vi "Color Matching.vi"() -> ()   [LabVIEW 2014]
doc: "This example shows how to use IMAQ ColorMatch to check LEDs on the front panel of an instrument. This example compares the color inside each region of interest (ROI) that surrounds an LED to the color spectrum of the expected color. The VI uses another example to learn the color spectrums."
uses:
  <vilib>/vision/NI_Vision_Development_Module.lvlib
panel:
  in  "Stop":bool
  out "Expected Pattern":T1
  out "Pass/Fail":T2
  in  "Orange Color Array":u32[][](array[colorbox])=[[14251822, 15569449, 16163116, 16492861, 15505723, 14721096, 14458954, 14263380, 14134114, 13741935, 13546876, 13746316, 14207641, 14539441, 13355173], [16488515, 16227377, 16163374, 16625472, 15902529, 15972181, 15775833, 15514209, 15253100, 14663027, 14401406, 14600845, 15259037, 15854523, 14078888], [16357434, 16293942, 15900982, 15574075, 15575618, 14328890, 14394944, 14527565, 14463835, 14201958, 14006129, 14336385, 14863504, 13813911, 14077859], [15634981, 16361273, 15903040, 14523444, 14525240, 14658112, 14527557, 14659921, 14858593, 14793838, 14597496, 14861446, 15322258, 14536867, 15393208], [15637012, 16494389, 16365383, 15315266, 15317058, 15118924, 14790476, 14659668, 14660961, 14661741, 14530424, 14596993, 14794891, 13681048, 14668464], [16756504, 15903782, 15051057, 14593334, 14529588, 14922316, 14527819, 14264912, 14462814, 14464110, 14530425, 14662277, 14925709, 14996142, 14010023], [16163605, 15442980, 14393902, 14529592, 14334002, 14265926, 14003015, 13871694, 14069083, 14135143, 14267253, 14728070, 15319954, 14534051, 14272166], [16163860, 15377187, 14130730, 14002480, 13412901, 14331972, 14069060, 14003533, 14135128, 14069861, 14201457, 14530943, 14991755, 14007703, 14338212], [16032531, 15706152, 14787891, 14462263, 13872171, 14463809, 14331972, 14201164, 14398553, 14267491, 14070892, 14399865, 14729349, 14600604, 15127724], [16032532, 15969326, 15313724, 15184961, 14528820, 14529087, 14397761, 14332746, 14399321, 14399588, 14202989, 14335353, 14664578, 14929567, 15062184], [16032795, 15968560, 15246650, 14986301, 14264621, 14265918, 14134593, 14135371, 14333274, 14268774, 14203506, 14401661, 14730889, 14469016, 14272668], [15834913, 15770930, 15114553, 14919995, 14263595, 14264898, 14002756, 14003534, 14136157, 14137196, 14138489, 14402439, 14797714, 14864293, 14799531], [15768871, 16033338, 15508544, 15576898, 14986802, 14659151, 14396496, 14331994, 14399080, 14400119, 14466949, 14665876, 15192480, 15456182, 15654335], [15965997, 16296256, 15705923, 15708484, 15183668, 15251037, 14988383, 14792295, 14793588, 14663554, 14730640, 15126176, 15587501, 14600620, 15061947], [14516283, 15768133, 16493647, 16561234, 16167503, 14856808, 14922862, 15056509, 15189902, 14928280, 14272669, 14142373, 14274989, 12501671, 11580573]]
  in  "Red Color Array":u32[][](array[colorbox])=[[12910680, 13959787, 15404161, 16651920, 16717199, 16650119, 16385925, 15992448, 16061061, 16329616, 16269977, 15948193, 16415413, 16750539, 15770563], [14225000, 15076985, 16061062, 16651407, 16716171, 16386947, 16453001, 16059268, 15996549, 16132749, 15678608, 15158677, 15296673, 15958452, 16032967], [15406707, 16127876, 16388746, 16453515, 16322183, 16059009, 16718994, 16588176, 16721812, 16726941, 16665503, 16079777, 16019626, 16417974, 15703489], [16128123, 16718219, 16585614, 16454287, 16323982, 16258957, 15932815, 15999119, 16329877, 16727453, 16403871, 15883168, 15690661, 15890860, 15505083], [16718470, 16718994, 16718232, 16653466, 16590240, 16592035, 16728495, 16729007, 16731058, 16734389, 16737205, 16739507, 16545972, 16417207, 15437750], [16652939, 16718746, 16719009, 16524711, 16396974, 16333232, 15942063, 16073902, 16403119, 16667569, 16670643, 16477107, 16151989, 15891638, 15173295], [16389775, 16653214, 16720811, 16593334, 16268989, 15811516, 16077760, 16274880, 16669121, 16736448, 16739780, 16743625, 16746443, 16747978, 15238577], [16390806, 16720551, 16723897, 16728519, 16600524, 16011465, 16342989, 16539851, 16539590, 16540354, 16607938, 16676804, 16417222, 16221381, 15961786], [16191618, 16654236, 16726711, 16730560, 16601794, 16735945, 16735693, 16736204, 16736711, 16475331, 16215231, 16086977, 16221381, 16354761, 16361936], [16717714, 16720294, 16726206, 16466885, 16075203, 16535750, 16538054, 16669636, 16670659, 16541376, 16346815, 16415682, 16484294, 16617674, 14913207], [16322191, 16719017, 16726216, 16730835, 16733142, 16735451, 16406977, 16538562, 16670913, 16606398, 16345786, 16217274, 16219323, 16155580, 15371705], [16586125, 16719781, 16725181, 16466117, 16401862, 16732365, 16669891, 16736196, 16737473, 16739009, 16740541, 16611260, 16482235, 16483516, 15371191], [16456322, 16721051, 16724654, 16333234, 16268722, 16730300, 15550127, 15813553, 16143025, 16276404, 16213170, 16084659, 16086964, 16022965, 15240119], [15799920, 16654988, 16724644, 16660395, 16726955, 16729779, 16732863, 16734146, 16735682, 16737473, 16739775, 16676542, 16482238, 16352959, 15505344], [15209577, 15997828, 16591004, 16395169, 16066202, 16656797, 16006064, 16072622, 16074415, 15879853, 15488939, 15229611, 15035821, 14972079, 14981823]]
  in  "Green Color Array":u32[][](array[colorbox])=[[5534475, 8890654, 10009630, 10535962, 10536465, 9812224, 9218821, 9415686, 9612811, 9809426, 9809179, 9873705, 9873205, 10069565, 10265687], [8562206, 10076183, 10405390, 9878533, 9351424, 9219584, 9482498, 9942279, 10337037, 10665238, 10664737, 10532138, 10136626, 10004021, 10200145], [9879321, 10209026, 10668801, 10338305, 9745152, 10337289, 9877506, 10403080, 10929426, 11257626, 11388710, 11321907, 10794807, 10399030, 10266189], [10340626, 9814272, 10471168, 10337792, 9744896, 10731021, 10469389, 11061012, 11455770, 11783971, 12046642, 12243009, 11847495, 11320134, 10792533], [10538258, 9616640, 10207232, 10008320, 9546496, 10467073, 10666519, 11257886, 11586851, 11783467, 12243516, 12703055, 12439383, 11845973, 10792282], [9880075, 9747712, 10469640, 10731275, 10796038, 11650829, 10797602, 11455018, 11717936, 11849012, 12374855, 12965979, 12636261, 11911519, 11120996], [10274581, 10470418, 10731796, 10533646, 10466819, 11124482, 11192111, 11849271, 12178236, 12309059, 12769108, 13360233, 12964975, 12174186, 12173688], [10733841, 10338567, 10074633, 10073101, 10007049, 10336267, 10336804, 11060273, 11783743, 12046665, 12243796, 12309086, 12111204, 11716195, 11583857], [10010883, 9812480, 9810944, 9678594, 10073095, 11059216, 11454766, 11717683, 11980859, 12112194, 12440656, 12703327, 12571238, 12242022, 12306810], [10274308, 10602240, 10732549, 10205443, 10269954, 10993163, 11257890, 11455015, 11652397, 11783478, 12046149, 12308819, 12110939, 11584344, 12306810], [10537738, 10799872, 10798592, 10599938, 10532864, 10730243, 11521052, 11981349, 12507442, 12704318, 12835403, 12900696, 12637024, 12176223, 11779955], [10405653, 9747712, 9614336, 10336256, 10730243, 10992388, 10008064, 10599948, 11126041, 11125540, 11124785, 11255873, 11320910, 11254868, 11714166], [10076451, 10207497, 10272000, 10664963, 10663682, 10531584, 10928653, 11257365, 11322909, 11125029, 11190068, 11649867, 12043869, 12175206, 11450230], [8693794, 10733341, 11587354, 11256336, 10465793, 10399488, 10204931, 10204679, 10072590, 10137883, 10597680, 10991686, 10925139, 10529878, 9476189], [6324746, 9614357, 11389212, 10795533, 10399748, 11385616, 9809152, 9743105, 9808651, 10334240, 11123004, 11253838, 10331982, 9147461, 7172414]]
  in  "Black Color Array":u32[][](array[colorbox])=[[66055, 66055, 66055, 66055, 66055, 66055, 66055, 66055, 66055, 66055, 66055, 66055, 66055, 66055, 66054], [65803, 65803, 65803, 65803, 65803, 65803, 66055, 66055, 66055, 66055, 66055, 66055, 66055, 66055, 66054], [65803, 65803, 65803, 65803, 65803, 65803, 66055, 66055, 66055, 66055, 66055, 66055, 66055, 66055, 66054], [65803, 65803, 65803, 65803, 65803, 65803, 66055, 66055, 66055, 66055, 66055, 66055, 66055, 66055, 66054], [65801, 65801, 65801, 65801, 65801, 65801, 66055, 66055, 66055, 66055, 66055, 66055, 66055, 66055, 66054], [65801, 65801, 65801, 65801, 65801, 65801, 66055, 66055, 66055, 66055, 66055, 66055, 66055, 66055, 66054], [65803, 65803, 65803, 65803, 65803, 65803, 66055, 66055, 66055, 66055, 66055, 66055, 66055, 66055, 66054], [65803, 65803, 65803, 65803, 65803, 65803, 66055, 66055, 66055, 66055, 66055, 66055, 66055, 66055, 66054], [65803, 65803, 65803, 65803, 65803, 65803, 66055, 66055, 66055, 66055, 66055, 66055, 66055, 66055, 66054], [66055, 66055, 66055, 66055, 66055, 66055, 66306, 66306, 66306, 66306, 66306, 66306, 66306, 66306, 66306], [66055, 66055, 66055, 66055, 66055, 66055, 66306, 66306, 66306, 66306, 66306, 66306, 66306, 66306, 66306], [65801, 65801, 65801, 65801, 65801, 65801, 66306, 66306, 66306, 66306, 66306, 66306, 66306, 66306, 66306], [131594, 131594, 131594, 131594, 131594, 131594, 66052, 66052, 66052, 66052, 66052, 66052, 66052, 66052, 66306], [131596, 131596, 131596, 131596, 131596, 131596, 66052, 66052, 66052, 66052, 66052, 66052, 66052, 66052, 66306], [197389, 197389, 197389, 197389, 197389, 197389, 66054, 66054, 66054, 66054, 66054, 66054, 66054, 66054, 66306]]
  out "Color Image":T3(plugin-control)
  out "Orange Color Spectrum":dbl[][](graph)
  out "Red Color Spectrum":dbl[][](graph)
  in  "Delay (s.)":dbl(slide)=0.9859154929577465 scale=0.0..3.0
  out "Black Color Spectrum":dbl[][](graph)
  out "Global Status":bool=TRUE
  out "Green Color Spectrum":dbl[][](graph)
  # "Overview: Demonstrates how to use the IMAQ Color Learn function to create a color spectrum array which is used by the IMAQ ColorMatch function to verify the LED has the expected color.\nRequirements: Vision Development Software.\nInstructions:  Run the VI."
  # "Faults"
  # "Inhibits"
  # "Limits"
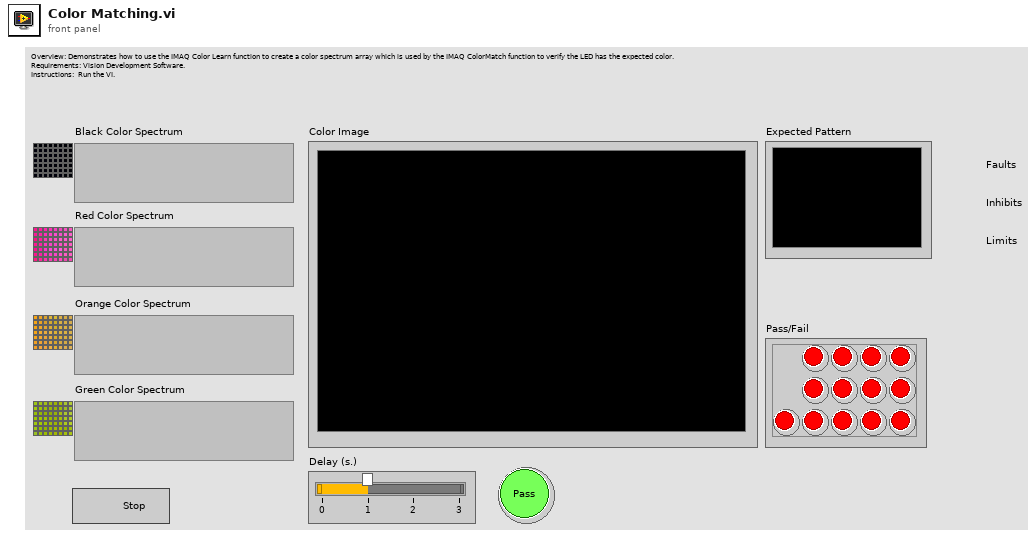
[diagram p1: front panel]
types:
  T1 = cluster{"on/off":i32, "Fault 1":i32, "Fault 2":i32, "Fault 3":i32, "Fault 4":i32, "Inhibit 1":i32, "Inhibit 2":i32, "Inhibit 3":i32, "Inhibit 4":i32, "Limit 1":i32, "Limit 2":i32, "Limit 3":i32, "Limit 4":i32}
  T2 = cluster{"Fault 2":bool, "Fault 1":bool, "Fault 3":bool, "Fault 4":bool, "Fault 5":bool, "Fault 6":bool, "Fault 7":bool, "Fault 8":bool, "Fault 9":bool, "Fault 10":bool, "Fault 11":bool, "Fault 12":bool, "Fault 13":bool}
  T3 = typedef "IMAQ Image.ctl" = refnum<image>
  T4 = cluster{"Global Rectangle":i32[], "Contours":cluster{"ID":enum32{"External", "Internal"}, "Type":u32, "Coordinates":i32[]}[]}[]
  T5 = cluster{"on/off":i32, "Fault 1":i32, "Fault 2":i32, "Fault 3":i32, "Fault 4":i32, "Inhibit 1":i32, "Inhibit 2":i32, "Inhibit 3":i32, "Inhibit 4":i32, "Limit 1":i32, "Limit 2":i32, "Limit 3":i32, "Limit 4":i32}[]
  T6 = typedef "Image Type" = u32
  T7 = cluster{"Desired Font (Application)":enum16{"User-specified Font", "Application Font", "System Font", "Dialog Font"}, "[User-specified Font]":cluster{"Font Name":string, "Size":i16, "Strikeout?":bool, "Italic?":bool, "Underline?":bool, "Outline?":bool, "Shadow?":bool, "Bold?":bool, "Rotation Angle":dbl}, "Horizontal Alignment":i16, "Vertical Alignment":i16}
  T8 = cluster{"Global Rectangle[0]":i32, "Global Rectangle[1]":i32}
  T9 = cluster{"[0]":bool, "[1]":bool, "[2]":bool, "[3]":bool, "[4]":bool, "[5]":bool, "[6]":bool, "[7]":bool, "[8]":bool, "[9]":bool, "[10]":bool, "[11]":bool, "[12]":bool}
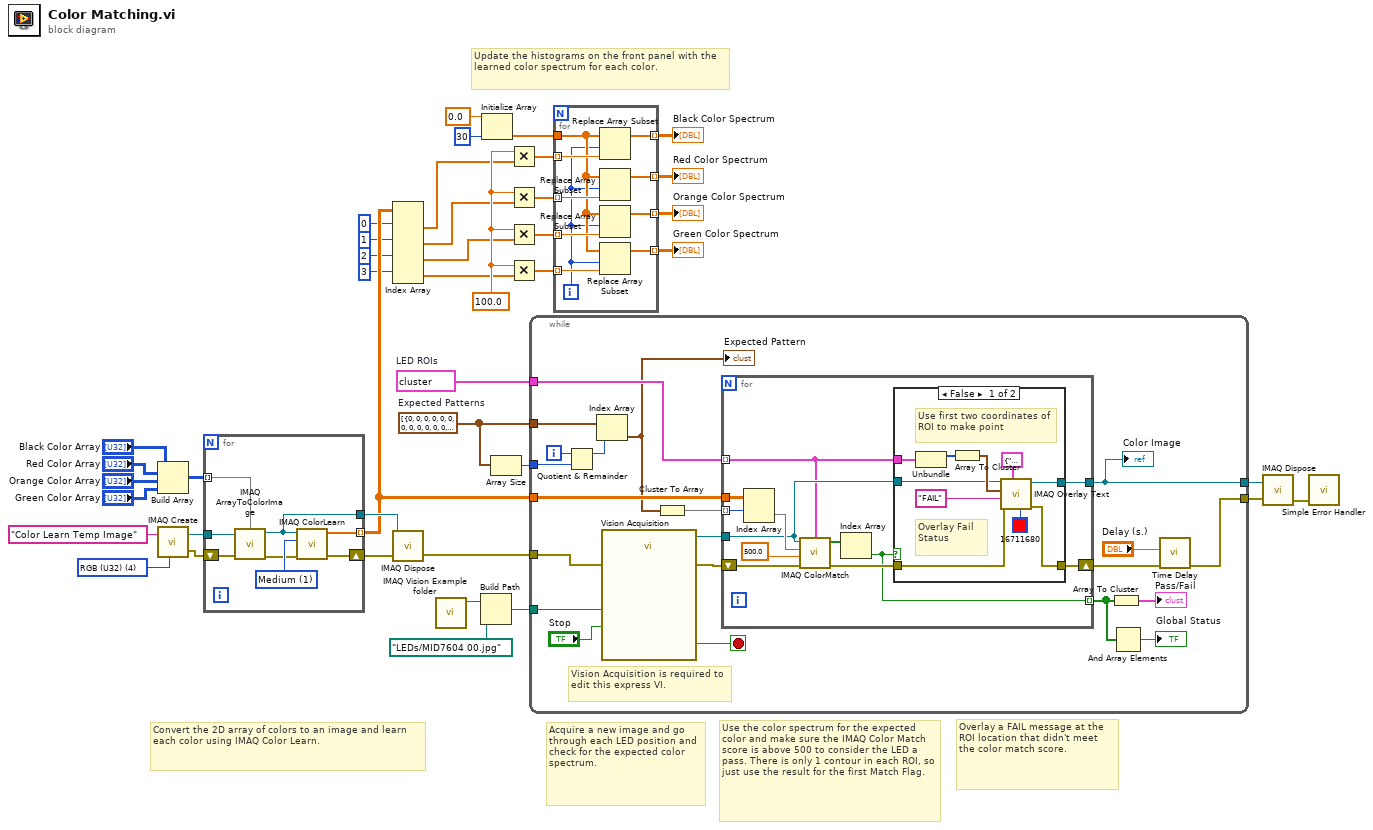
[diagram p0: block diagram]
diagram:
  w12 = T4 [{"Global Rectangle"=[32, 224, 53, 245], "Contours"=[{"ID"=enum."External", "Type"=3, "Coordinates"=[32, 224, 53, 245]}]}, {"Global Rectangle"=[86, 154, 98, 166], "Contours"=[{"ID"=enum."External", "Type"=3, "Coordinates"=[86, 154, 98, 166]}]}, {"Global Rectangle"=[136, 153, 149, 167], "Contours"=[{"ID"=enum."External", "Type"=3, "Coordinates"=[136, 153, 149, 167]}]}, {"Global Rectangle"=[188, 152, 200, 167], "Contours"=[{"ID"=enum."External", "Type"=3, "Coordinates"=[188, 152, 200, 167]}]}, {"Global Rectangle"=[236, 152, 250, 168], "Contours"=[{"ID"=enum."External", "Type"=3, "Coordinates"=[236, 152, 250, 168]}]}, {"Global Rectangle"=[87, 194, 99, 207], "Contours"=[{"ID"=enum."External", "Type"=3, "Coordinates"=[87, 194, 99, 207]}]}, {"Global Rectangle"=[136, 193, 149, 208], "Contours"=[{"ID"=enum."External", "Type"=3, "Coordinates"=[136, 193, 149, 208]}]}, {"Global Rectangle"=[189, 193, 201, 207], "Contours"=[{"ID"=enum."External", "Type"=3, "Coordinates"=[189, 193, 201, 207]}]}, {"Global Rectangle"=[236, 194, 250, 208], "Contours"=[{"ID"=enum."External", "Type"=3, "Coordinates"=[236, 194, 250, 208]}]}, {"Global Rectangle"=[86, 233, 100, 246], "Contours"=[{"ID"=enum."External", "Type"=3, "Coordinates"=[86, 233, 100, 246]}]}, {"Global Rectangle"=[135, 233, 150, 246], "Contours"=[{"ID"=enum."External", "Type"=3, "Coordinates"=[135, 233, 150, 246]}]}, {"Global Rectangle"=[187, 232, 201, 248], "Contours"=[{"ID"=enum."External", "Type"=3, "Coordinates"=[187, 232, 201, 248]}]}, {"Global Rectangle"=[236, 232, 250, 247], "Contours"=[{"ID"=enum."External", "Type"=3, "Coordinates"=[236, 232, 250, 247]}]}]  # LED ROIs
  w14 = T5 [{"on/off"=0, "Fault 1"=0, "Fault 2"=0, "Fault 3"=0, "Fault 4"=0, "Inhibit 1"=0, "Inhibit 2"=0, "Inhibit 3"=0, "Inhibit 4"=0, "Limit 1"=0, "Limit 2"=0, "Limit 3"=0, "Limit 4"=0}, {"on/off"=3, "Fault 1"=1, "Fault 2"=1, "Fault 3"=1, "Fault 4"=1, "Inhibit 1"=2, "Inhibit 2"=2, "Inhibit 3"=2, "Inhibit 4"=2, "Limit 1"=3, "Limit 2"=3, "Limit 3"=3, "Limit 4"=3}, {"on/off"=3, "Fault 1"=1, "Fault 2"=1, "Fault 3"=1, "Fault 4"=1, "Inhibit 1"=0, "Inhibit 2"=0, "Inhibit 3"=0, "Inhibit 4"=2, "Limit 1"=3, "Limit 2"=3, "Limit 3"=3, "Limit 4"=3}, {"on/off"=3, "Fault 1"=0, "Fault 2"=0, "Fault 3"=0, "Fault 4"=0, "Inhibit 1"=0, "Inhibit 2"=0, "Inhibit 3"=0, "Inhibit 4"=0, "Limit 1"=3, "Limit 2"=3, "Limit 3"=3, "Limit 4"=3}, {"on/off"=3, "Fault 1"=0, "Fault 2"=0, "Fault 3"=0, "Fault 4"=0, "Inhibit 1"=0, "Inhibit 2"=0, "Inhibit 3"=0, "Inhibit 4"=0, "Limit 1"=0, "Limit 2"=0, "Limit 3"=0, "Limit 4"=0}, {"on/off"=3, "Fault 1"=0, "Fault 2"=0, "Fault 3"=0, "Fault 4"=0, "Inhibit 1"=0, "Inhibit 2"=0, "Inhibit 3"=0, "Inhibit 4"=0, "Limit 1"=3, "Limit 2"=0, "Limit 3"=0, "Limit 4"=0}, {"on/off"=3, "Fault 1"=0, "Fault 2"=0, "Fault 3"=0, "Fault 4"=0, "Inhibit 1"=0, "Inhibit 2"=0, "Inhibit 3"=0, "Inhibit 4"=0, "Limit 1"=0, "Limit 2"=3, "Limit 3"=0, "Limit 4"=0}, {"on/off"=3, "Fault 1"=0, "Fault 2"=0, "Fault 3"=0, "Fault 4"=0, "Inhibit 1"=0, "Inhibit 2"=0, "Inhibit 3"=0, "Inhibit 4"=0, "Limit 1"=0, "Limit 2"=0, "Limit 3"=3, "Limit 4"=0}, {"on/off"=3, "Fault 1"=0, "Fault 2"=0, "Fault 3"=0, "Fault 4"=0, "Inhibit 1"=0, "Inhibit 2"=0, "Inhibit 3"=0, "Inhibit 4"=0, "Limit 1"=0, "Limit 2"=0, "Limit 3"=0, "Limit 4"=3}, {"on/off"=3, "Fault 1"=0, "Fault 2"=1, "Fault 3"=0, "Fault 4"=0, "Inhibit 1"=0, "Inhibit 2"=0, "Inhibit 3"=0, "Inhibit 4"=0, "Limit 1"=0, "Limit 2"=0, "Limit 3"=0, "Limit 4"=0}, {"on/off"=3, "Fault 1"=0, "Fault 2"=0, "Fault 3"=1, "Fault 4"=0, "Inhibit 1"=0, "Inhibit 2"=0, "Inhibit 3"=0, "Inhibit 4"=0, "Limit 1"=0, "Limit 2"=0, "Limit 3"=0, "Limit 4"=0}, {"on/off"=3, "Fault 1"=0, "Fault 2"=0, "Fault 3"=0, "Fault 4"=1, "Inhibit 1"=0, "Inhibit 2"=0, "Inhibit 3"=0, "Inhibit 4"=0, "Limit 1"=0, "Limit 2"=0, "Limit 3"=0, "Limit 4"=0}, {"on/off"=3, "Fault 1"=0, "Fault 2"=0, "Fault 3"=0, "Fault 4"=0, "Inhibit 1"=0, "Inhibit 2"=2, "Inhibit 3"=2, "Inhibit 4"=0, "Limit 1"=0, "Limit 2"=0, "Limit 3"=0, "Limit 4"=3}, {"on/off"=3, "Fault 1"=1, "Fault 2"=0, "Fault 3"=0, "Fault 4"=0, "Inhibit 1"=0, "Inhibit 2"=0, "Inhibit 3"=0, "Inhibit 4"=2, "Limit 1"=0, "Limit 2"=3, "Limit 3"=3, "Limit 4"=0}, {"on/off"=3, "Fault 1"=0, "Fault 2"=0, "Fault 3"=1, "Fault 4"=1, "Inhibit 1"=2, "Inhibit 2"=2, "Inhibit 3"=0, "Inhibit 4"=0, "Limit 1"=0, "Limit 2"=0, "Limit 3"=3, "Limit 4"=3}, {"on/off"=3, "Fault 1"=1, "Fault 2"=0, "Fault 3"=0, "Fault 4"=0, "Inhibit 1"=0, "Inhibit 2"=0, "Inhibit 3"=0, "Inhibit 4"=2, "Limit 1"=3, "Limit 2"=3, "Limit 3"=3, "Limit 4"=0}, {"on/off"=3, "Fault 1"=0, "Fault 2"=0, "Fault 3"=0, "Fault 4"=1, "Inhibit 1"=0, "Inhibit 2"=2, "Inhibit 3"=0, "Inhibit 4"=2, "Limit 1"=3, "Limit 2"=0, "Limit 3"=3, "Limit 4"=0}]  # Expected Patterns
  w6 = T6 4 items=["Grayscale (U8)", "Grayscale (I16)", "Grayscale (SGL)", "Complex (CSG)", "RGB (U32)", "HSL (U32)", "RGB (U64)", "Grayscale (U16)"] ("Image Type")
  w42 = 100.0
  # "Overlay a FAIL message at the ROI location that didn't meet the color match score."
  # "Acquire a new image and go through each LED position and check for the expected color spectrum."
  # "Update the histograms on the front panel with the learned color spectrum for each color."
  # "Convert the 2D array of colors to an image and learn each color using IMAQ Color Learn."
  # "Use the color spectrum for the expected color and make sure the IMAQ Color Match score is above 500 to consider the LED a pass. There is only 1 contour in each ROI, so just use the result for the first Match Flag."
  n1 = Build Array("Black Color Array", "Red Color Array", "Orange Color Array", "Green Color Array") -> (w30:u32[][][])
  n2 = call "IMAQ Create"("Image Name"="Color Learn Temp Image", "Image Type"=w6) -> ("New Image"=w28:T3, "error out"=w27:errorcluster)  [unwired: 3 in]
  n3 = for {
    tunnel: w28 -> [w50]
    tunnel: w30 -> [w44] mode=indexing
    tunnel: [w47] -> w16 mode=indexing
    shift-right: [w46] -> w22
    shift-left: w27 -> [w49]
    tunnel: [w45] -> w21
    w48 = u32 1 items=["Low", "Medium", "High"] ("Color Sensitivity")
    n4 = call "IMAQ ArrayToColorImage"("Image Pixels (U32)"=w44, "Image"=w50, "error in (no error)"=w49) -> ("Image Out"=w45:T3, "error out"=w43:errorcluster)  [unwired: 2 in]
    n5 = call "IMAQ ColorLearn"("Image"=w45, "Color Sensitivity"=w48, "error in (no error)"=w43) -> ("Color Spectrum"=w47:dbl[], "error out"=w46:errorcluster)  [unwired: 5 in]
  }
  n6 = Index Array(array=w16, index (row) #1=0 ("index (row)"), index (row) #2=1 ("index (row)"), index (row) #3=2 ("index (row)"), index (row) #4=3 ("index (row)")) -> (element #1=w26:dbl[], element #2=w25:dbl[], element #3=w24:dbl[], element #4=w23:dbl[])  [unwired: 4 in]
  n7 = call "IMAQ Dispose"("Image"=w21, "error in (no error)"=w22) -> ("error out"=w17:errorcluster)  [unwired: 4 in]
  n8 = call "IMAQ Vision Example folder.vi"() -> ("Example Image Path"=w19:path)  [unwired: 11 in]
  n9 = Build Path(base path=w19, name or relative path=path "LEDs/MID7604 00.jpg") -> (appended path=w18:path)
  n10 = Initialize Array(0.0 ("Element Data"), 30) -> (w36:dbl[])
  n11 = Array Size(array=w14) -> (size(s)=w13:i32)
  n12 = Multiply(x=w42, y=w26) -> (x*y=w38:dbl[])
  n13 = Multiply(x=w42, y=w25) -> (x*y=w39:dbl[])
  n14 = Multiply(x=w42, y=w24) -> (x*y=w40:dbl[])
  n15 = Multiply(x=w42, y=w23) -> (x*y=w41:dbl[])
  n16 = while {
    tunnel: w18 -> [w70]
    tunnel: w17 -> [w69]
    tunnel: w16 -> [w66]
    tunnel: [w64] -> w15
    tunnel: w14 -> [w61]
    tunnel: w13 -> [w60]
    tunnel: w12 -> [w59]
    tunnel: [w55] -> w11
    i -> [w68]
    stop <- w58 stop-if-true
    # "Vision Acquisition is required to edit this express VI."
    n17 = Quotient & Remainder(x=w68, y=w60) -> (x-y*floor(x/y)=w71:i32)  [unwired: 1 out]
    n18 = Index Array(array=w61, index=w71) -> (element=w51:T1)
    "Expected Pattern" <- w51
    n19 = call "Vision Acquisition"("Image Path"=w70, "Stop (F)"="Stop", "error in"=w69) -> ("Image Out"=w65:T3, "Stopped"=w58:bool, "error out"=w52:errorcluster)  [unwired: 22 in]
    n20 = Cluster To Array(cluster=w51) -> (array=w67:i32[])
    n21 = for {
      tunnel: w66 -> [w83]
      tunnel: w65 -> [w78]
      tunnel: w59 -> [w77] mode=indexing
      tunnel: w67 -> [w80] mode=indexing
      tunnel: [w74] -> w64
      tunnel: [w73] -> w63 mode=indexing
      shift-right: [w72] -> w56
      shift-left: w52 -> [w76]
      n22 = Index Array(array=w83, index (row)=w80) -> (element=w82:dbl[])  [unwired: 1 in]
      n23 = call "IMAQ ColorMatch"("ROI Descriptor"=w77, "Image"=w78, "Color Spectrum"=w82, "Minimum Match Score"=500.0, "error in (no error)"=w76) -> ("Match Flag"=w79:bool[], "error out"=w75:errorcluster)  [unwired: 1 in, 2 out]
      n24 = Index Array(array=w79) -> (element=w73:bool)  [unwired: 1 in]
      n25 = case shown="False" w73 {
        tunnel: w78 -> [w86 w95]
        tunnel: w77 -> [w90 _]
        tunnel: w75 -> [w85 w94]
        tunnel: [w91 w95] -> w74
        tunnel: [w84 w94] -> w72
        frame False {
          # "Overlay Fail Status"
          # "Use first two coordinates of ROI to make point"
          n26 = Unbundle(w90) -> ("Global Rectangle"=w89:i32[])  [unwired: 1 out]
          n27 = Array To Cluster(array=w89) -> (cluster=w88:T8)
          n28 = call "IMAQ Overlay Text"("BG Color (Transparent)"=u32 16711680, "Font, Size & Style"=T7 {"Desired Font (Application)"=enum."Application Font", "[User-specified Font]"={"Font Name"="", "Size"=12, "Strikeout?"=FALSE, "Italic?"=FALSE, "Underline?"=FALSE, "Outline?"=FALSE, "Shadow?"=FALSE, "Bold?"=FALSE, "Rotation Angle"=0.0}, "Horizontal Alignment"=0, "Vertical Alignment"=1}, "error in (no error)"=w85, "String"="FAIL", "Origin"=w88, "Image"=w86) -> ("error out"=w84:errorcluster, "Image Out"=w91:T3)  [unwired: 4 in]
        }
        frame True {
          # "Color Matches"
        }
      }
    }
    "Color Image" <- w64
    n29 = Array To Cluster(array=w63) -> (cluster=→"Pass/Fail":T9)
    n30 = And Array Elements(Boolean array=w63) -> (logical AND=→"Global Status":bool)
    n31 = call "Time Delay"("error in (no error)"=w56, "Delay Time (s)"="Delay (s.)") -> ("error out"=w55:errorcluster)  [unwired: 9 in]
  }
  n32 = for {
    tunnel: w41 -> [w102] mode=indexing
    tunnel: w40 -> [w103] mode=indexing
    tunnel: w39 -> [w104] mode=indexing
    tunnel: w38 -> [w105] mode=indexing
    tunnel: [w99] -> w37 mode=indexing
    tunnel: [w98] -> w33 mode=indexing
    tunnel: [w97] -> w32 mode=indexing
    tunnel: [w96] -> w31 mode=indexing
    tunnel: w36 -> [w101]
    i -> [w100]
    n33 = Replace Array Subset(array=w101, new element=w105, index=w100) -> (w99:dbl[])
    n34 = Replace Array Subset(array=w101, new element=w104, index=w100) -> (w98:dbl[])
    n35 = Replace Array Subset(array=w101, new element=w103, index=w100) -> (w97:dbl[])
    n36 = Replace Array Subset(array=w101, new element=w102, index=w100) -> (w96:dbl[])
  }
  "Black Color Spectrum" <- w37
  "Red Color Spectrum" <- w33
  "Orange Color Spectrum" <- w32
  "Green Color Spectrum" <- w31
  n37 = call "IMAQ Dispose"("Image"=w15, "error in (no error)"=w11) -> ("error out"=w1:errorcluster)  [unwired: 1 in, 3 out]
  n38 = call <vilib>:"Simple Error Handler.vi"("error in (no error)"=w1) -> ()  [unwired: 4 in, 5 out]
